vi "Change Mode.vi"(8 "error in (no error)":errorcluster, 10 "Editing Mode":enum32{"Default Mode", "Advanced Mode"}(radio), 11 "Numeric Data Type in":refnum<class "Numeric Data Type.lvclass">) -> (0 "error out":errorcluster, 3 "Numeric Data Type out":refnum<class "Numeric Data Type.lvclass">)   [LabVIEW 2018, in "Numeric Data Type.lvclass"]
uses:
  Numeric Data Type.lvclass
  Numeric Data Type.lvclass/Numeric Data Type.ctl
  Reference Default-Advanced Tab.vi
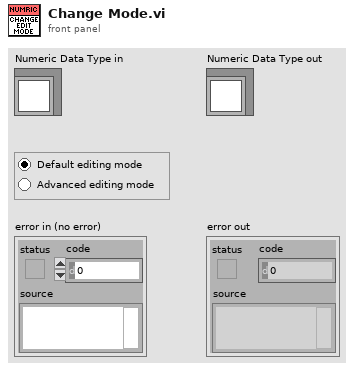
[diagram p1: front panel]
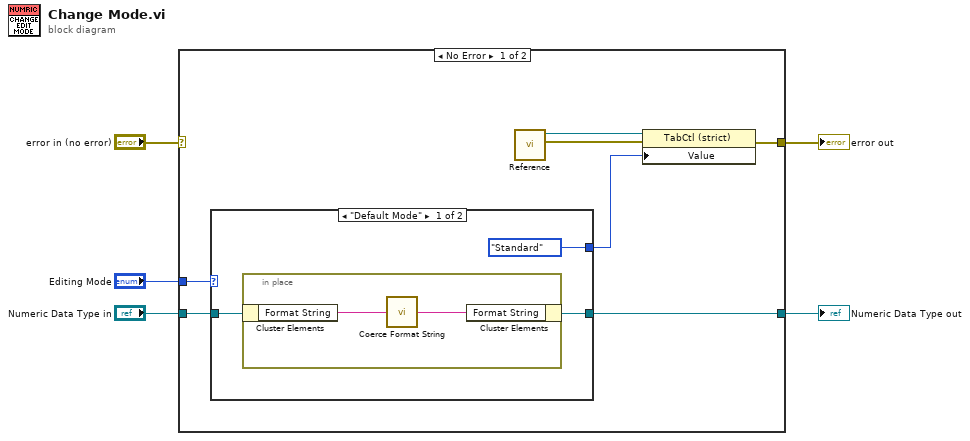
[diagram p0: block diagram]
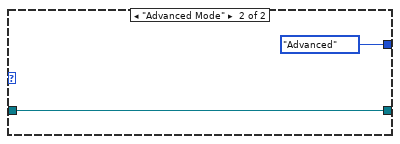
[diagram p2: hidden frame]
diagram:
  n1 = case shown="No Error" "error in (no error)" {
    selector: "error in (no error)" -> [_ w21]
    tunnel: [w8 w21] -> w4
    tunnel: [w10 w20] -> w2
    tunnel: "Numeric Data Type in" -> [w11 w20]
    tunnel: "Editing Mode" -> [w12 _]
    frame No Error {
      n2 = case shown="\"Default Mode\"" w12 {
        tunnel: w11 -> [w15 w19]
        tunnel: [w14 w19] -> w10
        tunnel: [enum32{"Standard", "Advanced"}."Standard" ("Value") enum32{"Standard", "Advanced"}."Advanced" ("Value")] -> w9
        frame "Default Mode" {
          n3 = in-place {
            n4 = in-place-cluster #1(w15) -> ("Format String"=w17:string)
            n5 = call "Coerce Format String.vi"("Format String"=w17) -> ("Coerced String"=w16:string)
            n6 = in-place-cluster #1("Format String"=w16) -> (w14:refnum<class "Numeric Data Type.lvclass">)
          }
        }
        frame "Advanced Mode" {
        }
      }
      n7 = call-poly "Reference.vi"() -> ("error out"=w6:errorcluster, "Default/Advanced Tab"=w7:refnum<vi>)  [unwired: 10 in]
      n8 = property class="TabCtl (strict)"(reference=w7, error in=w6, "Value"=w9) -> (error out=w8:errorcluster)  [unwired: 1 out]
    }
    frame Error {
    }
  }
  "error out" <- w4
  "Numeric Data Type out" <- w2
